vi "Actor Core.vi"(8 "error in":errorcluster, 11 "ATM Controller in":refnum<class "Sim User Console Actor.lvclass">) -> (0 "error out":errorcluster, 3 "Actor out":refnum<class "Actor.lvclass">)   [LabVIEW 2019, in "Sim User Console Actor.lvlib" / "Sim User Console Actor.lvclass"]
doc: "(<B>Filename</B>: Actor Framework.lvlib:Actor.lvclass:Actor Core.vi)\n\nReceives messages to the actor, reacts to them, and initiates any error handling that may shut the actor down.\n\nDescendant classes may override this VI to append parallel tasks for the actor to complete while it handles messages. Overrides use the Call Parent Method node."
uses:
  Sim User Console Actor.lvclass
  <vilib>/ActorFramework/Stop Msg/Stop Msg.lvclass
  <vilib>/ActorFramework/Actor/Actor.lvclass
  C:/Workspace/CLA/ATM AF 2nd/User Console Actor/User Console Actor/User Console Actor.lvclass
  C:/Program Files (x86)/National Instruments/LabVIEW 2019/vi.lib/ActorFramework/Actor/Actor.lvclass
  ATM Controller/ATM Controller Messages/Set Transaction Msg/Set Transaction Msg.lvclass
  ATM Controller/ATM Controller Messages/Set Card Read Msg/Set Card Read Msg.lvclass
  ATM Controller/ATM Controller Messages/Set State Msg/Set State Msg.lvclass
  ATM Controller/ATM Controller/State -Enum.ctl
  ATM Controller/ATM Controller/ATM Controller.lvclass
  ATM Controller/ATM Controller Messages/Set Timer Msg/Set Timer Msg.lvclass
  ATM Controller/ATM Controller Messages/Get Keypad Msg/Get Keypad Msg.lvclass
  User Console Actor/User Console Actor/User Console Actor.lvclass
  Keypad - Cluster.ctl
  Transactions -Cluster.ctl
panel:
  in  "Card Reader":bool
  in  "Transactions":T1
  in  "Keypad":T2
  # "[Covers: UI1]\n[Covers: UI2] \n[Covers: UI2A] \n[Covers: UI2B]\n[Covers: UI2C]"
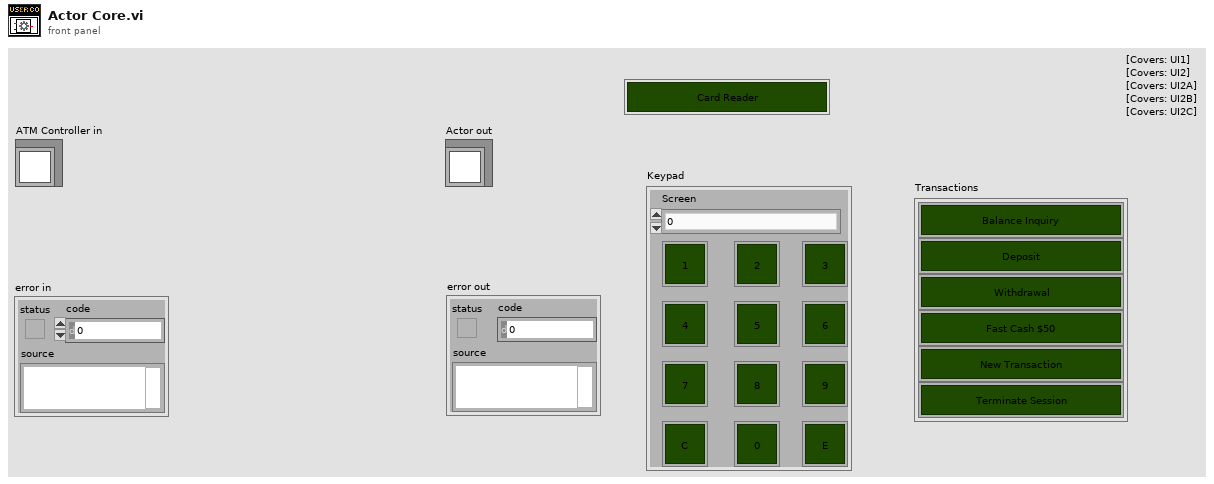
[diagram p1: front panel]
types:
  T1 = typedef "Sim User Console Actor.lvlib/Sim User Console Actor.lvclass/Transactions -Cluster.ctl" = cluster{"Balance Inquiry":bool, "Deposit":bool, "Withdrawal":bool, "Fast Cash $50":bool, "New Transaction":bool, "Terminate Session":bool}
  T2 = typedef "Sim User Console Actor.lvlib/Sim User Console Actor.lvclass/Keypad - Cluster.ctl" = cluster{"1":bool, "1 2":bool, "1 3":bool, "1 4":bool, "1 5":bool, "1 6":bool, "1 7":bool, "1 8":bool, "1 9":bool, "C":bool, "1 11":bool, "E":bool, "Screen":dbl}
  T3 = typedef "ATM Controller.lvlib/ATM Controller.lvclass/State -Enum.ctl" = enum16{"Initial", "Idle", "Login", "Balance Inquiry", "Deposit", "Withdrawal", "Fast Cash", "Terminate", "Inactivity Timeout"}
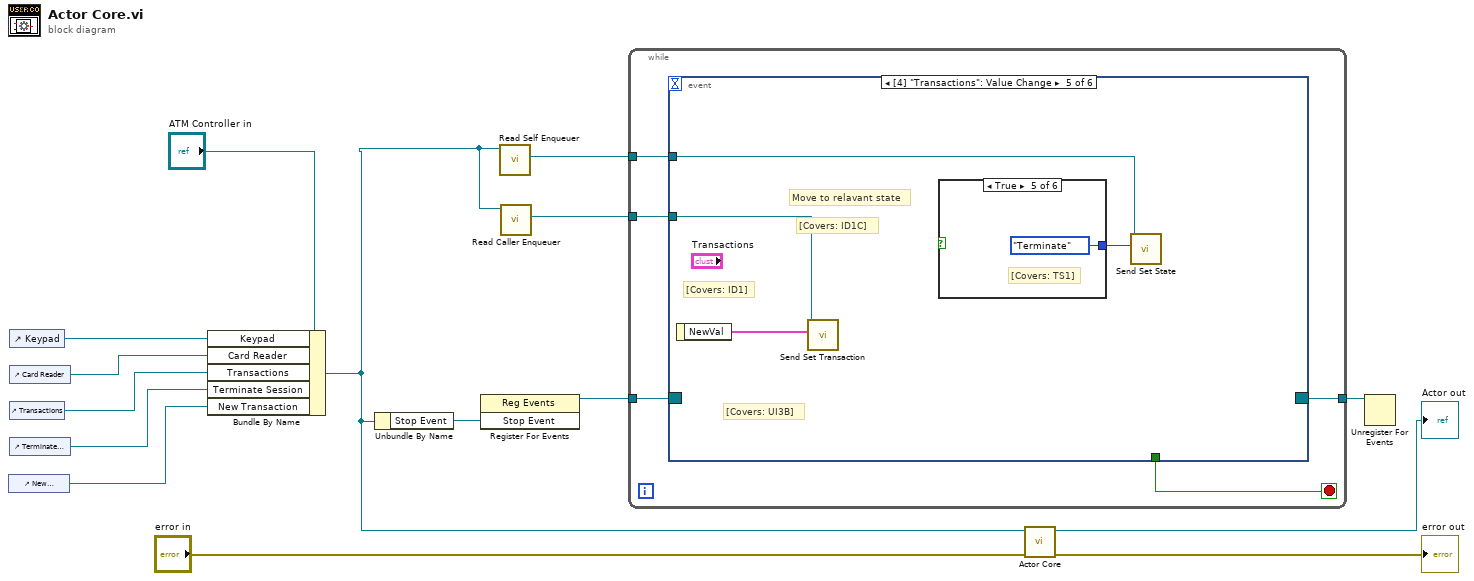
[diagram p0: block diagram]
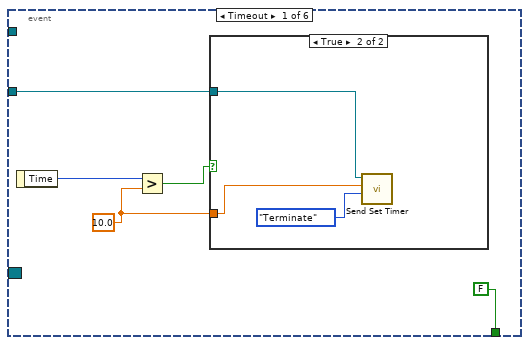
[diagram p2: hidden frame]
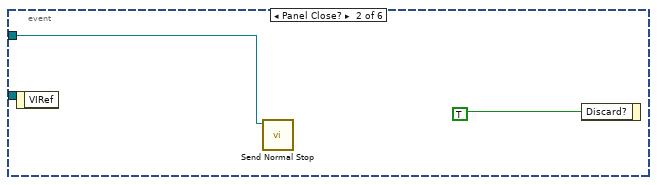
[diagram p4: hidden frame]
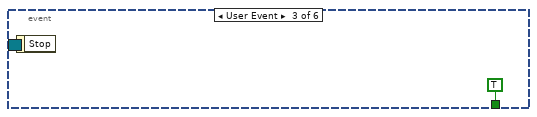
[diagram p5: hidden frame]
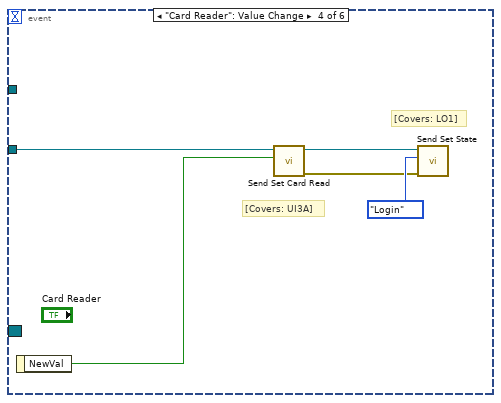
[diagram p6: hidden frame]
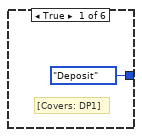
[diagram p7: hidden frame]
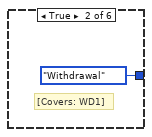
[diagram p8: hidden frame]
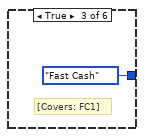
[diagram p9: hidden frame]
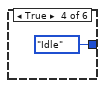
[diagram p10: hidden frame]
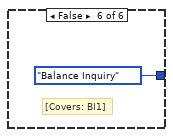
[diagram p11: hidden frame]
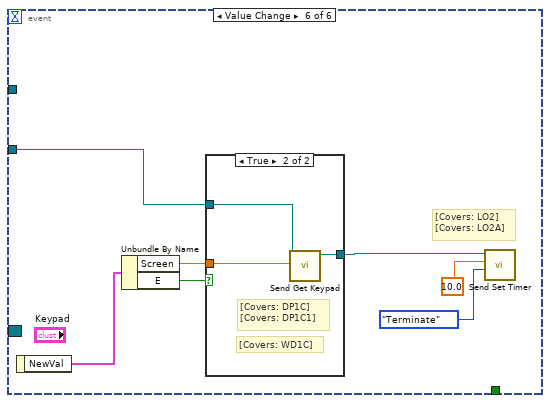
[diagram p12: hidden frame]
diagram:
  n1 = control-ref of="New Transaction"() -> (w1:refnum<vi>)
  n2 = control-ref of="Keypad"() -> (w6:refnum<vi>)
  n3 = control-ref of="Card Reader"() -> (w5:refnum<vi>)
  n4 = control-ref of="Transactions"() -> (w4:refnum<vi>)
  n5 = control-ref of="Terminate Session"() -> (w2:refnum<vi>)
  n6 = Bundle By Name(cluster="ATM Controller in", "Keypad"=w6, "Card Reader"=w5, "Transactions"=w4, "Terminate Session"=w2, "New Transaction"=w1) -> (w3:refnum<class "Sim User Console Actor.lvclass">)
  n7 = Unbundle By Name(w3) -> ("Stop Event"=w12:refnum<user-event>)
  n8 = register-events(w12) -> (reference out=w11:refnum<event-registration>)  [unwired: 2 in, 1 out]
  n9 = call <vilib>:"Read Self Enqueuer.vi"("Actor"=w3) -> ("Self Enqueuer"=w9:refnum<class "Message Enqueuer.lvclass">)  [unwired: 10 in]
  n10 = call <vilib>:"Read Caller Enqueuer.vi"("Actor"=w3) -> ("Caller Enqueuer"=w8:refnum<class "Message Enqueuer.lvclass">)  [unwired: 10 in]
  n11 = while {
    tunnel: w11 -> [w19]
    tunnel: [w18] -> w10
    tunnel: w9 -> [w17]
    tunnel: w8 -> [w16]
    stop <- w20 stop-if-true
    n12 = event shown="[4] \"Transactions\": Value Change" {
      selector: w19 -> [_ _ _ _ _ _]
      dyn-events: [_ _ _ _ _ _] -> w18
      timeout: _ -> [_ _ _ _ _ _]
      tunnel: [FALSE _ TRUE _ _ _] -> w20
      tunnel: w17 -> [_ w30 _ _ w38 _]
      tunnel: w16 -> [w21 _ _ w36 w40 w48]
      event Timeout {
        w23 = 10.0 ("Target time")
        n13 = event-data() -> ("Time"=w24:u32)  [unwired: 1 in]
        n14 = Greater?(x=w24, y=w23) -> (0:w22:bool)
        n15 = case shown="True" w22 {
          tunnel: w23 -> [_ w27]
          tunnel: w21 -> [_ w26]
          frame False {
          }
          frame True {
            n16 = call "Send Set Timer.vi"("State"=State_-Enum."Terminate", "Target time"=w27, "Message Enqueuer"=w26) -> ()  [unwired: 7 in, 2 out]
          }
        }
      }
      event Panel Close? {
        n17 = event-data() -> ()  [unwired: 1 in, 1 out]
        n18 = call <vilib>:"Send Normal Stop.vi"("Message Enqueuer"=w30) -> ()  [unwired: 10 in, 1 out]
        n19 = event-data("Discard?"=TRUE) -> ()  [unwired: 1 in, 1 out]
      }
      event User Event {
        n20 = event-data() -> ()  [unwired: 1 in, 1 out]
      }
      event "Card Reader": Value Change {
        # "[Covers: LO1]"
        # "[Covers: UI3A]"
        n21 = event-data() -> ("NewVal"=w35:bool)  [unwired: 1 in]
        n22 = call "Send Set Card Read.vi"("Card read"=w35, "Message Enqueuer"=w36) -> ("error out"=w32:errorcluster, "Message Enqueuer out"=w34:refnum<class "Message Enqueuer.lvclass">)  [unwired: 8 in]
        n23 = call "Send Set State.vi"("error in (no error)"=w32, "State"=State_-Enum."Login", "Message Enqueuer"=w34) -> ()  [unwired: 7 in, 2 out]
      }
      event Value Change {
        # "[Covers: ID1]"
        # "[Covers: ID1C]"
        # "Move to relavant state"
        # "[Covers: UI3B]"
        n24 = event-data() -> ("NewVal"=w39:T1)  [unwired: 1 in]
        n25 = call "Send Set Transaction.vi"("Transactions"=w39, "Message Enqueuer"=w40) -> ()  [unwired: 8 in, 2 out]
        n26 = case shown="\"Terminate Session\"" {
          selector: _ -> [_ _ _ _ _ _]
          tunnel: [State_-Enum."Deposit" ("State") State_-Enum."Withdrawal" ("State") State_-Enum."Fast Cash" ("State") State_-Enum."Idle" ("State") State_-Enum."Terminate" ("State") State_-Enum."Balance Inquiry" ("State")] -> w37
          frame True {
            # "[Covers: DP1]"
          }
          frame True {
            # "[Covers: WD1]"
          }
          frame True {
            # "[Covers: FC1]"
          }
          frame True {
          }
          frame True {
            # "[Covers: TS1]"
          }
          frame False {
            # "[Covers: BI1]"
          }
        }
        n27 = call "Send Set State.vi"("State"=w37, "Message Enqueuer"=w38) -> ()  [unwired: 8 in, 2 out]
      }
      event Value Change {
        # "[Covers: LO2]\n[Covers: LO2A]"
        n28 = event-data() -> ("NewVal"=w51:T2)  [unwired: 1 in]
        n29 = Unbundle By Name(w51) -> ("Screen"=w49:dbl, "E"=w50:bool)
        n30 = case shown="True" w50 {
          tunnel: w49 -> [_ w56]
          tunnel: w48 -> [w54 w57]
          tunnel: [w54 w55] -> w47
          frame False {
          }
          frame True {
            # "[Covers: WD1C]"
            # "[Covers: DP1C]\n[Covers: DP1C1]"
            n31 = call "Send Get Keypad.vi"("Keypad Screen"=w56, "Message Enqueuer"=w57) -> ("Message Enqueuer out"=w55:refnum<class "Message Enqueuer.lvclass">)  [unwired: 8 in, 1 out]
          }
        }
        n32 = call "Send Set Timer.vi"("State"=State_-Enum."Terminate", "Target time"=10.0, "Message Enqueuer"=w47) -> ()  [unwired: 7 in, 2 out]
      }
    }
  }
  n33 = call-parent "Actor Core.vi"("error in"="error in", "Actor in"=w3) -> ("error out"=→"error out":errorcluster, "Actor out"=→"Actor out":refnum<class "Actor.lvclass">)  [unwired: 8 in]
  n34 = Unregister For Events(event registration refnum=w10) -> ()  [unwired: 1 in, 1 out]
